vi "Assemble_Command.vi"(0 "Controller ID":string, 1 "Acceleration":dbl format="%#.6f", 2 "Target":dbl min=-210.0 max=109.0 step=0.001 format="%.3f", 3 "Step factor":dbl, 4 "Speed":dbl, 8 "Shutter? (F)":bool) -> (7 "command":string)   [LabVIEW 2012]
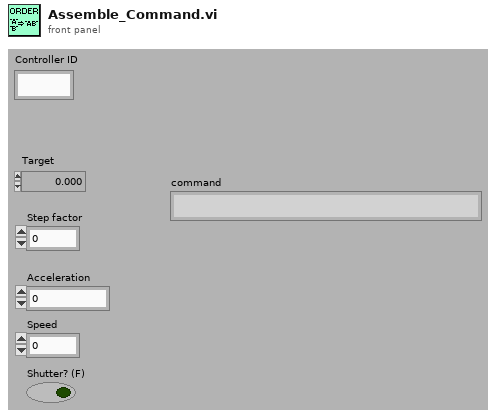
[diagram p1: front panel]
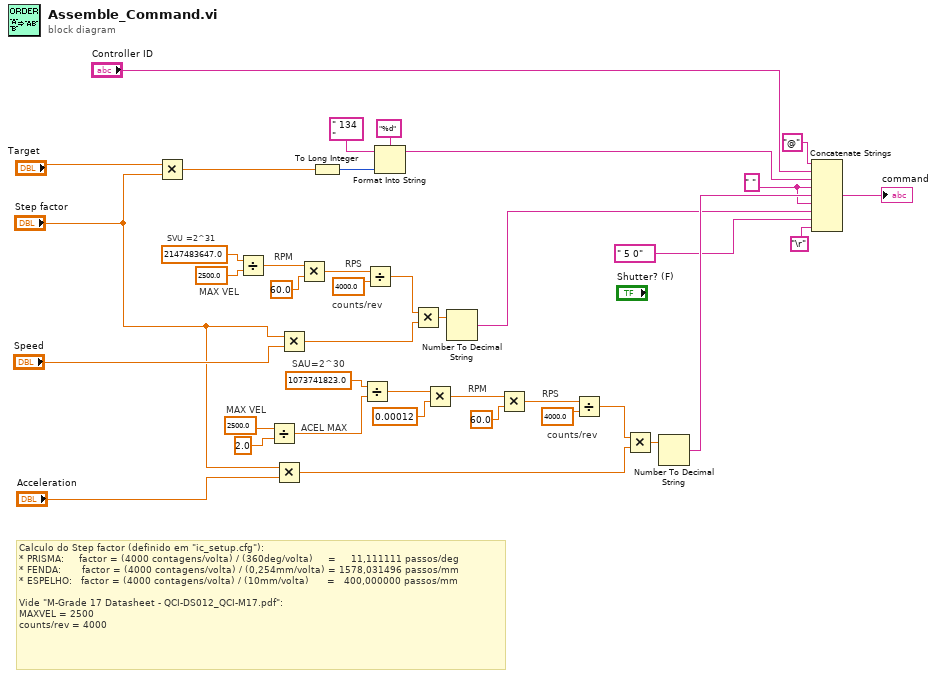
[diagram p0: block diagram]
diagram:
  w4 = " "
  # "Calculo do Step factor (definido em \"ic_setup.cfg\"):\n* PRISMA:     factor = (4000 contagens/volta) / (360deg/volta)     =     11,111111 passos/deg\n* FENDA:       factor = (4000 contagens/volta) / (0,254mm/volta) = 1578,031496 passos/mm\n* ESPELHO:   factor = (4000 contagens/volta) / (10mm/volta)      =   400,000000 passos/mm\n\nVide \"M-Grade 17 Datasheet - QCI-DS012_QCI-M17.pdf\":\nMAXVEL = 2500 \ncounts/rev = 4000"
  # "counts/rev"
  # "counts/rev"
  # "RPS"
  # "RPM"
  # "ACEL MAX"
  # "MAX VEL"
  # "SAU=2^30"
  # "RPS"
  # "MAX VEL"
  # "SVU =2^31"
  # "RPM"
  n1 = Multiply(x="Target", y="Step factor") -> (x*y=w2:dbl)
  n2 = Divide(x=2147483647.0 ("Numeric"), y=2500.0 ("Numeric")) -> (x/y=w28:dbl)
  n3 = Divide(x=2500.0 ("Numeric"), y=2.0) -> (x/y=w19:dbl)
  n4 = Multiply(x="Step factor", y="Acceleration") -> (x*y=w13:dbl)
  n5 = Multiply(x="Step factor", y="Speed") -> (x*y=w24:dbl)
  n6 = Multiply(x=w28, y=60.0) -> (x*y=w26:dbl)
  n7 = To Long Integer(number=w2) -> (32bit integer=w39:i32)
  n8 = Divide(x=1073741823.0 ("Numeric"), y=w19) -> (x/y=w17:dbl)
  n9 = Divide(x=w26, y=4000.0) -> (x/y=w23:dbl)
  n10 = Format Into String(format string="%d", initial string=" 134 ", w39) -> (resulting string=w33:string)  [unwired: 1 in, 1 out]
  n11 = Multiply(x=w23, y=w24) -> (x*y=w7:dbl)
  n12 = Multiply(x=w17, y=0.00012) -> (x*y=w15:dbl)
  n13 = Number To Decimal String(number=w7) -> (decimal integer string=w5:string)  [unwired: 1 out]
  n14 = Multiply(x=w15, y=60.0) -> (x*y=w11:dbl)
  n15 = Divide(x=w11, y=4000.0) -> (x/y=w12:dbl)
  n16 = Multiply(x=w12, y=w13) -> (x*y=w8:dbl)
  n17 = Number To Decimal String(number=w8) -> (decimal integer string=w6:string)  [unwired: 1 out]
  n18 = Concatenate Strings("@" ("string"), "Controller ID", w33, w4, w6, w4, w5, " 5 0", "\r") -> (→"command":string)
